vi "Chessy_Drive_Main.vi"(0 "Speed_Main":dbl, 1 "Turning_Main":dbl, 5 "Speed_Limit":dbl, 7 "Turning_Limit":dbl, 12 "Quick_Turn":bool) -> (3 "Left_Motor":dbl format="%.2f", 14 "Right_Motor":dbl format="%.2f")   [LabVIEW 2013]
panel:
  in  "Turning Scale":dbl=1.5
  in  "Turning Y":dbl[](array[numeric])=[-1.0, -0.5, -0.21, 0.0, 0.0, 0.0, 0.21, 0.5, 1.0]
  in  "Turning X":dbl[](array[numeric])=[-1.0, -0.75, -0.155, -0.15, 0.0, 0.15, 0.155, 0.75, 1.0]
  in  "Speed Y":dbl[](array[numeric])=[-1.0, -0.5, -0.21, 0.0, 0.0, 0.0, 0.21, 0.5, 1.0]
  in  "Speed X":dbl[](array[numeric])=[-1.0, -0.75, -0.155, -0.15, 0.0, 0.15, 0.155, 0.75, 1.0]
  in  "Turning_Hyd_Deadband":dbl=0.75
  in  "Speed_Hyd_Deadband":dbl=0.75
  out "Delta":dbl format="%.2f"
  # "Chessy Drive"
  # "This subystem takes turning and speed controls from a xbox joystick \nand creats left and right motor values"
  # "Tunning"
  # "Inputs"
  # "Test Points"
  # "Ouputs"
  # "Joystick Map (Lookup Table)"
  # "Hyp Cmd Deadband"
  # "Turning Power Mode"
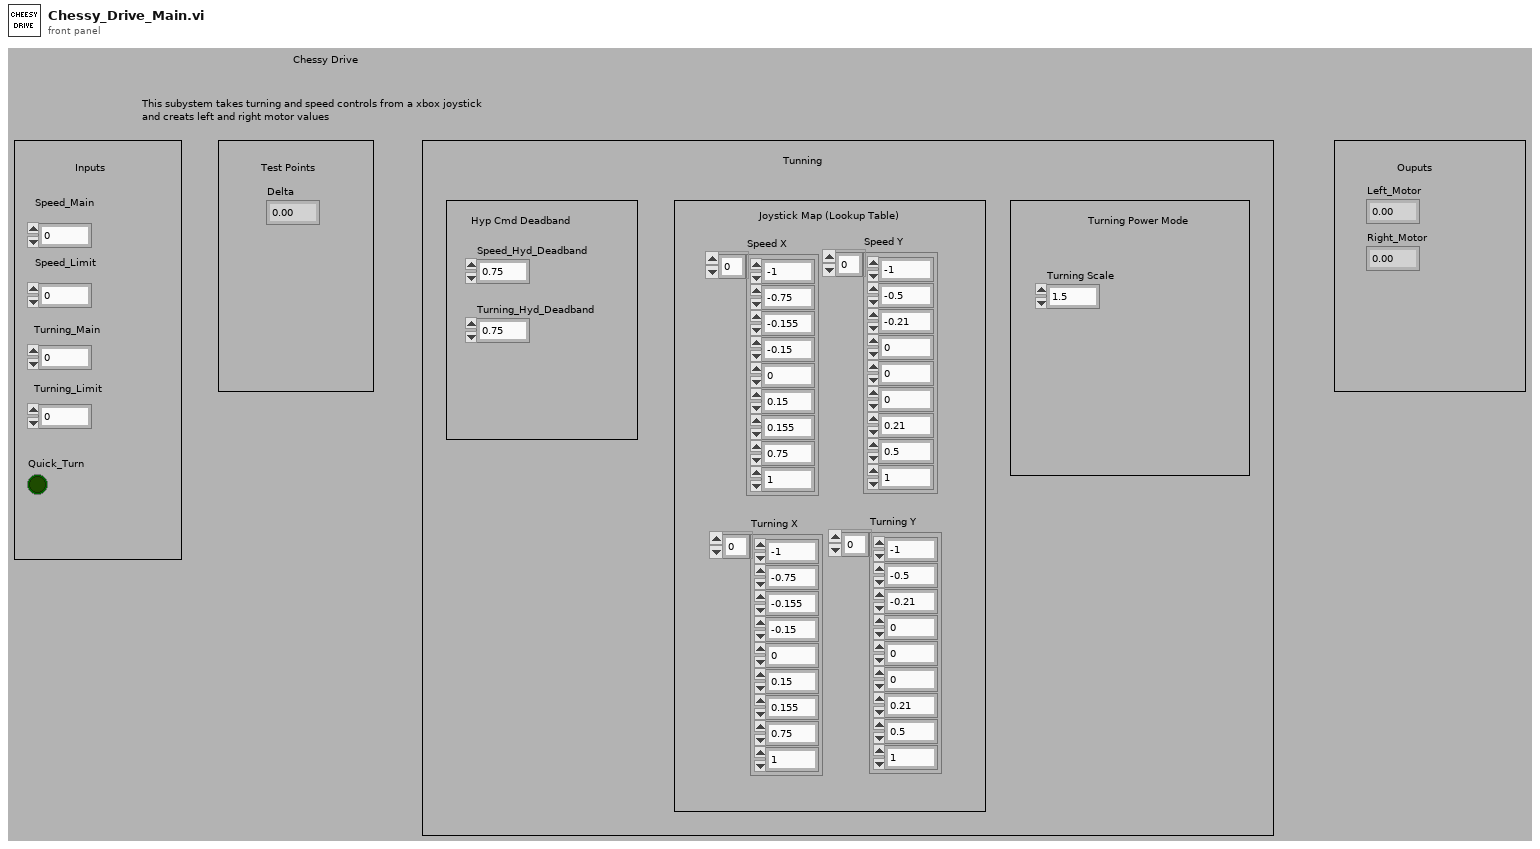
[diagram p1: front panel]
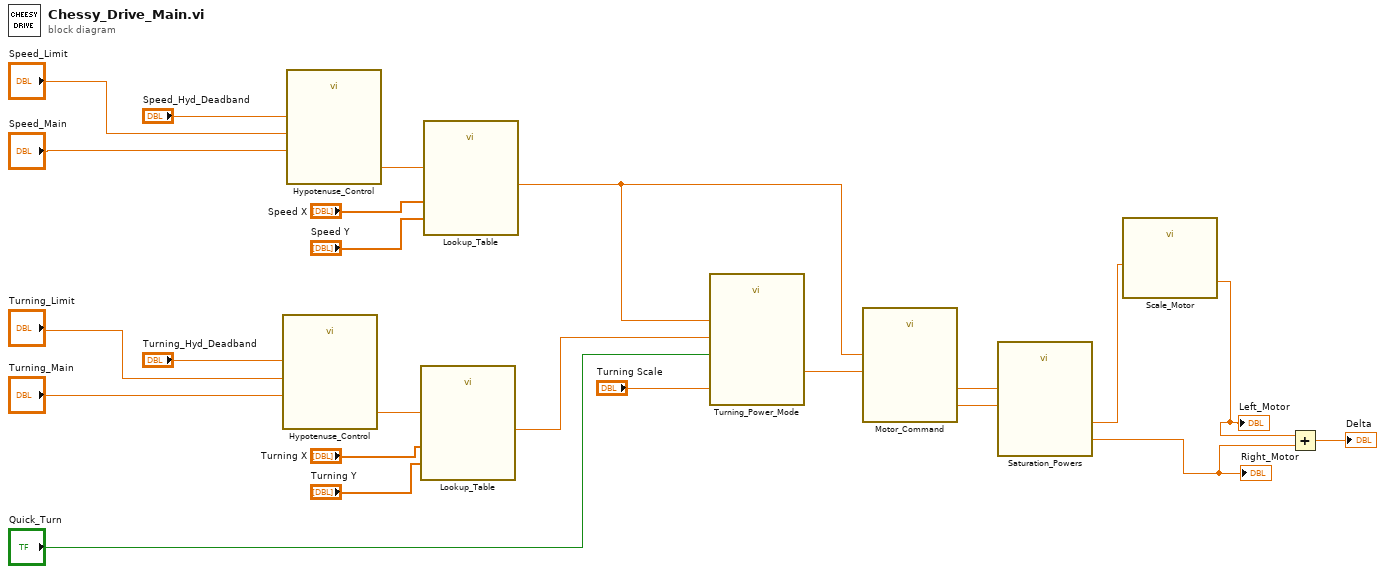
[diagram p0: block diagram]
diagram:
  n1 = call "Hypotenuse_Control.vi"("Deadband"="Turning_Hyd_Deadband", "Limit_Axis"="Turning_Limit", "Main_Axis"="Turning_Main") -> ("Axis_Adj"=w6:dbl)  [unwired: 8 in]
  n2 = call "Hypotenuse_Control.vi"("Deadband"="Speed_Hyd_Deadband", "Limit_Axis"="Speed_Limit", "Main_Axis"="Speed_Main") -> ("Axis_Adj"=w10:dbl)  [unwired: 8 in]
  n3 = call "Lookup_Table.vi"("Y_Array"="Turning Y", "x_in"=w6, "X_Array"="Turning X") -> ("y_out"=w16:dbl)  [unwired: 6 in]
  n4 = call "Lookup_Table.vi"("Y_Array"="Speed Y", "x_in"=w10, "X_Array"="Speed X") -> ("y_out"=w17:dbl)  [unwired: 6 in]
  n5 = call "Turning_Power_Mode.vi"("Turning_Scale"="Turning Scale", "Quick_Turn"="Quick_Turn", "Turning"=w16, "Power"=w17) -> ("Turning_Correction"=w19:dbl)  [unwired: 7 in]
  n6 = call "Motor_Command.vi"("Turning"=w19, "Power"=w17) -> ("Right_Motor"=w22:dbl, "Left_Motor"=w20:dbl)  [unwired: 8 in]
  n7 = call "Saturation_Powers.vi"("Right_Motor"=w22, "Left_Motor"=w20) -> ("Right_Motor_Say"=w18:dbl, "Left_Motor_Sat"=w2:dbl)  [unwired: 8 in]
  "Right_Motor" <- w18
  n8 = call "Scale_Motor.vi"("Input"=w2) -> ("Output"=w1:dbl)  [unwired: 10 in]
  "Left_Motor" <- w1
  n9 = Add(x=w1, y=w18) -> (x+y=→"Delta":dbl)
